vi "Untitled 1.vi"() -> ()   [LabVIEW 2011]
panel:
  out "data":variant
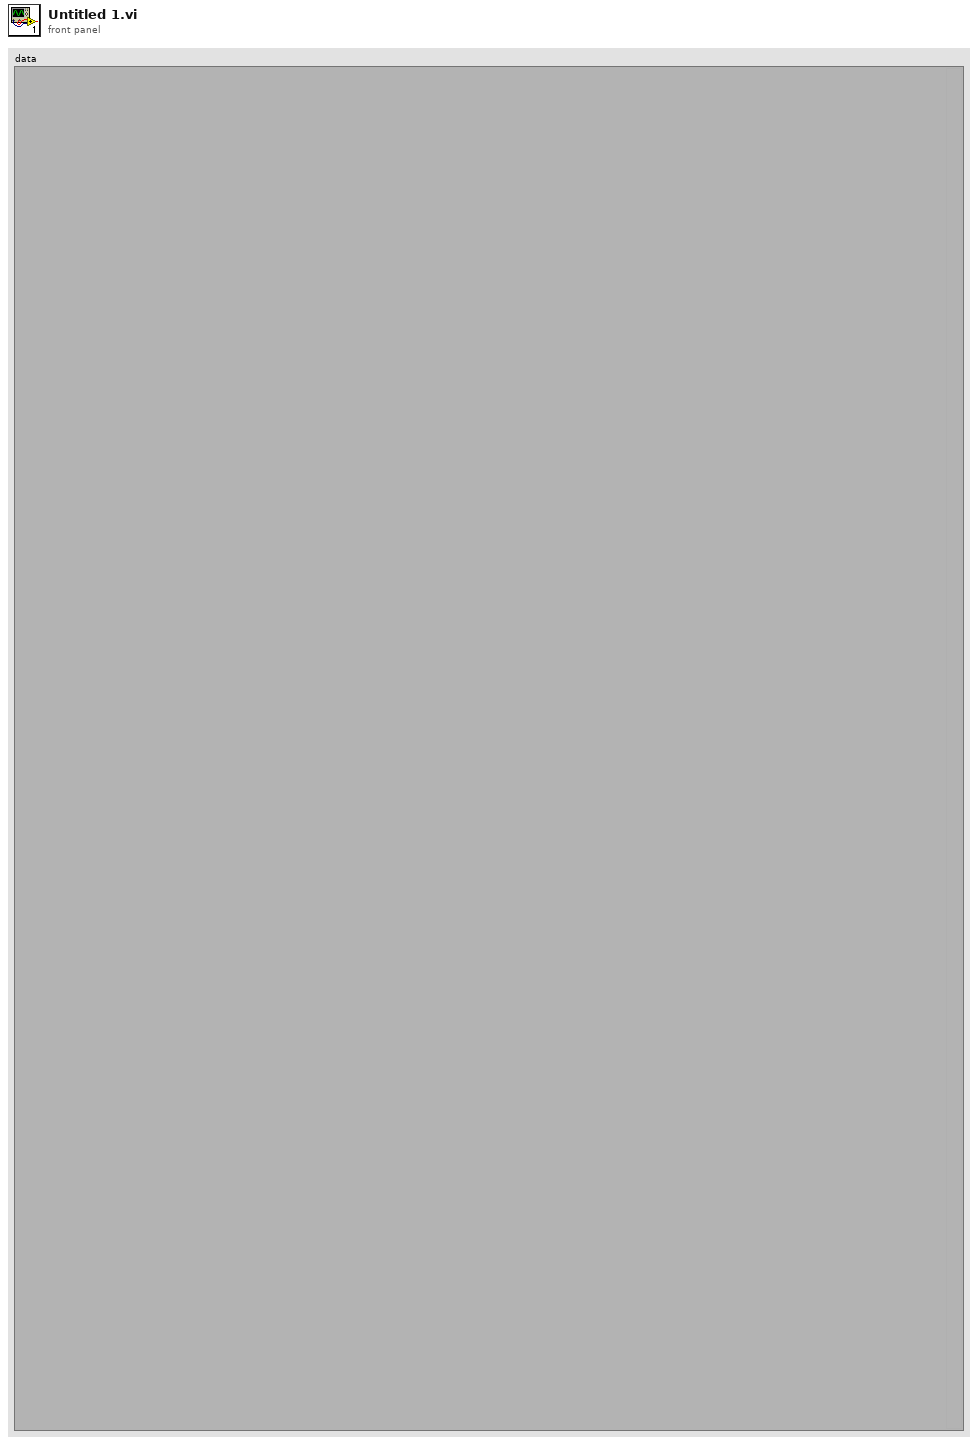
[diagram p1: front panel]
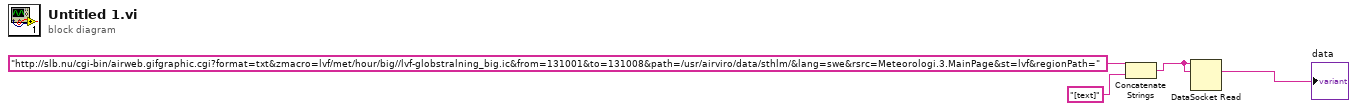
[diagram p0: block diagram]
diagram:
  n1 = Concatenate Strings("http://slb.nu/cgi-bin/airweb.gifgraphic.cgi?format=txt&zmacro=lvf/met/hour/big//lvf-globstralning_big.ic&from=131001&to=131008&path=/usr/airviro/data/sthlm/&lang=swe&rsrc=Meteorologi.3.MainPage&st=lvf&regionPath=" ("connection in"), "[text]" ("string")) -> (w1:string)
  n2 = DataSocket Read(10:w1, 11:w1) -> (2:→"data":string)  [unwired: 3 in, 6 out]
